vi "GetPlotBndsInScreenCoord.vi"(8 "error in (no error)":errorcluster, 10 "IntensityGraph in":refnum<vi>, 11 "VI in":refnum<vi>) -> (0 "error out":errorcluster, 1 "Bounds Screen Coordinates":T1, 3 "IntensityGraph out":refnum<vi>)   [LabVIEW 2023]
doc: "This VI finds out the intensity graph's plot area bounds and translates them into screen position."
uses:
  <vilib>/Utility/miscctls.llb/LVRectTypeDef.ctl
  <vilib>/Utility/miscctls.llb/LVPositionTypeDef.ctl
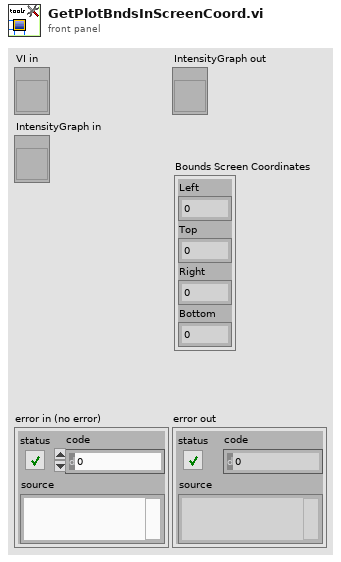
[diagram p1: front panel]
types:
  T1 = typedef "LVRectTypeDef.ctl" = cluster{"Left":i16, "Top":i16, "Right":i16, "Bottom":i16}
  T2 = typedef "LVPositionTypeDef.ctl" = cluster{"Left":i32, "Top":i32}
  T3 = typedef "LVPointTypeDef.ctl" = cluster{"Horizontal":i16, "Vertical":i16}
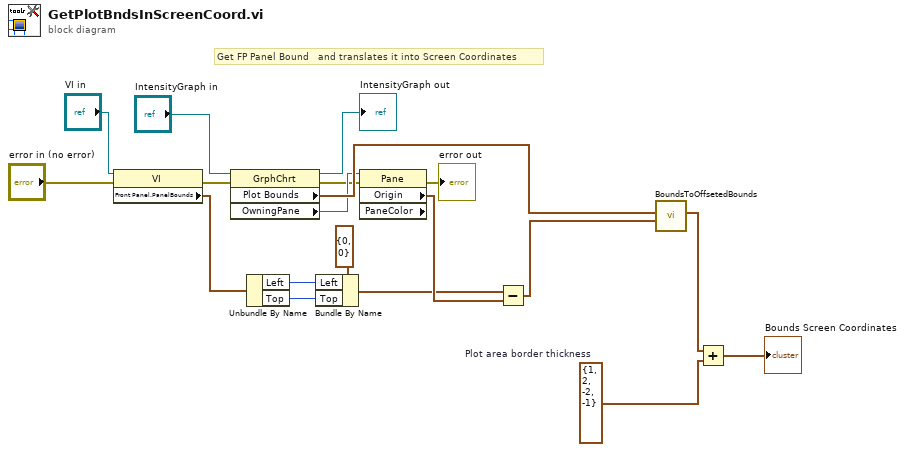
[diagram p0: block diagram]
diagram:
  w2 = T1 {"Left"=1, "Top"=2, "Right"=-2, "Bottom"=-1}  # Plot area border thickness
  # "Get FP Panel Bound   and translates it into Screen Coordinates"
  n1 = property on="Property Node" class="VI"(reference="VI in", error in="error in (no error)") -> (error out=w7:errorcluster, "Front Panel.PanelBounds"=w19:T1)  [unwired: 1 out]
  n2 = property on="Property Node" class="GrphChrt"(reference="IntensityGraph in", error in=w7) -> (reference out=→"IntensityGraph out":refnum<vi>, error out=w6:errorcluster, "Plot Bounds"=w12:T1, "OwningPane"=w9:refnum<vi>)
  n3 = Unbundle By Name(w19) -> ("Left"=w16:i16, "Top"=w17:i16)
  n4 = Bundle By Name(cluster=T2 {"Left"=0, "Top"=0} ("Position"), "Left"=w16, "Top"=w17) -> (w4:T2)
  n5 = property on="Property Node" class="Pane" props=["Origin", "PaneColor"](reference=w9, error in=w6) -> (error out=→"error out":errorcluster, "Origin"=w10:T3)  [unwired: 2 out]
  n6 = Subtract(x=w4, y=w10) -> (x-y=w11:T2)
  n7 = call "BoundsToOffsetedBounds.vi"("Offset"=w11, "Bounds"=w12) -> ("Bounds + Offset"=w3:T1)  [unwired: 9 in]
  n8 = Add(x=w3, y=w2) -> (x+y=→"Bounds Screen Coordinates":T1)
